vi "Driver Add.vi"(8 "error in (no error)":errorcluster, 10 "Driver Record":T1, 11 "Connection Refnum":T2) -> (0 "error out":errorcluster, 2 "New Driver Record":T1, 3 "Connection Refnum":T2)   [LabVIEW 2011]
uses:
  Driver Record.ctl
  SI.LIB/ODBC/SQL Controls/Connection Refnum.ctl
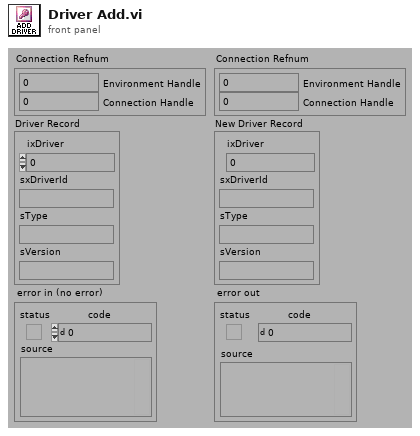
[diagram p1: front panel]
types:
  T1 = typedef "Driver Record.ctl" = cluster{"ixDriver":i32, "sxDriverId":string, "sType":string, "sVersion":string}
  T2 = typedef "Connection Refnum.ctl" = cluster{"Environment Handle":i32, "Connection Handle":i32}
  T3 = typedef "Statement Refnum.ctl" = cluster{"Statement Handle":i32, "Parameter Number":u16}
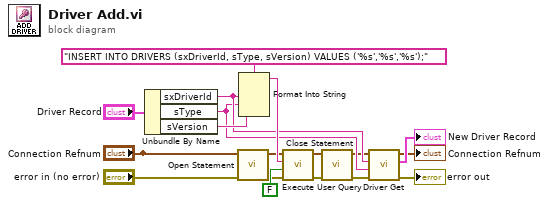
[diagram p0: block diagram]
diagram:
  n1 = Unbundle By Name("Driver Record") -> ("sxDriverId"=w6:string, "sType"=w5:string, "sVersion"=w7:string)
  n2 = call "Open Statement.vi"("error in (no error)"="error in (no error)", "Connection Refnum"="Connection Refnum") -> ("error out"=w12:errorcluster, "Statement Refnum"=w11:T3)  [unwired: 4 out]
  n3 = Format Into String(format string="INSERT INTO DRIVERS (sxDriverId, sType, sVersion) VALUES ('%s','%s','%s');" ("User Query"), w6, w5, w7) -> (resulting string=w16:string)  [unwired: 2 in, 1 out]
  n4 = call "Execute User Query.vi"("error in (no error)"=w12, "Return Data? (f)"=FALSE, "User Query"=w16, "Statement Refnum"=w11) -> ("error out"=w13:errorcluster, "Statement Refnum"=w14:T3)  [unwired: 2 out]
  n5 = call "Close Statement.vi"("error in (no error)"=w13, "Statement Refnum"=w14) -> ("error out"=w9:errorcluster)  [unwired: 5 out]
  n6 = call "Driver Get.vi"("error in (no error)"=w9, "sType"=w5, "sxDriverId"=w6, "Connection Refnum"="Connection Refnum") -> ("error out"=→"error out":errorcluster, "Driver Record"=→"New Driver Record":T1, "Connection Refnum"=→"Connection Refnum":T2)  [unwired: 5 out]
